vi "标定等待面板.vi"() -> ()   [LabVIEW 2013]
panel:
  in  "LVDT2ZADC":i64
  in  "LVDT2FADC":i64
  in  "LVDT1FADC":i64
  in  "LVDT1ZADC":i64
  in  "stop":bool
  # "标定中......"
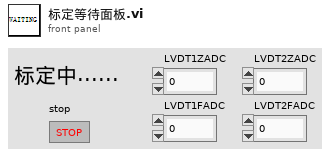
[diagram p1: front panel]
types:
  T1 = enum32{"DEH零度标定", "DEH满度标定", "阀门满度标定", "阀门零度标定", "最大正输出标定", "最大负输出标定", "零输出输出标定", "表头20mA标定", "表头4mA标定", "稳态偏差校准", "阀门位置自动标定", "转速4mA标定", "转速20mA标定"}
  T2 = cluster{"联机状态":bool, "外置清零信号":bool, "卡件工作模式":enum16{"无输出", "正常工作", "阀门常开", "阀门常闭"}, "卡件序列号":string, "卡件物理地址":string, "伺服阀输出电流CH1":dbl, "输出通道状态CH1":bool, "伺服阀输出电流CH2":dbl, "输出通道状态CH2":bool, "伺服输出使能CH1 ":bool, "伺服输出使能CH2":bool, "LVDT1类型":enum16{"未接入", "直流", "交流"}, "LVDT1直流回路":bool, "LVDT1次级线圈 2":bool, "LVDT1次级线圈 1":bool, "LVDT1初级线圈":bool, "LVDT2类型":enum16{"未接入", "直流", "交流"}, "LVDT2直流回路":bool, "LVDT2次级线圈 2":bool, "LVDT2次级线圈 1":bool, "LVDT2初级线圈":bool, "DEH回路状态":bool, "DEH类型":enum16{"内置", "外接"}, "转速反馈使能":bool, "LVDT1信号采样百分比":dbl, "LVDT2信号采样百分比":dbl, "DEH指令值":u8, "转速差反馈量":dbl, "回路1转速":dbl, "回路2转速":dbl, "回路3转速":dbl, "中选转速":dbl, "LVDT1 ADC":i16, "LVDT2 ADC":i16, "DEH ADC":i16, "LVDT1ZADC":i16, "LVDT2ZADC":i16, "LVDT1FADC":i16, "LVDT2FADC":i16, "DehZeroCali":bool, "DehFullCali":bool, "LVDT1ZeroCali":bool, "LVDT1FullCali":bool, "LVDT2ZeroCali":bool, "LVDT2FullCali":bool, "转速零度标定":i16, "转速满度标定":i16, "转速指令采样值":i16, "标准转速":dbl}
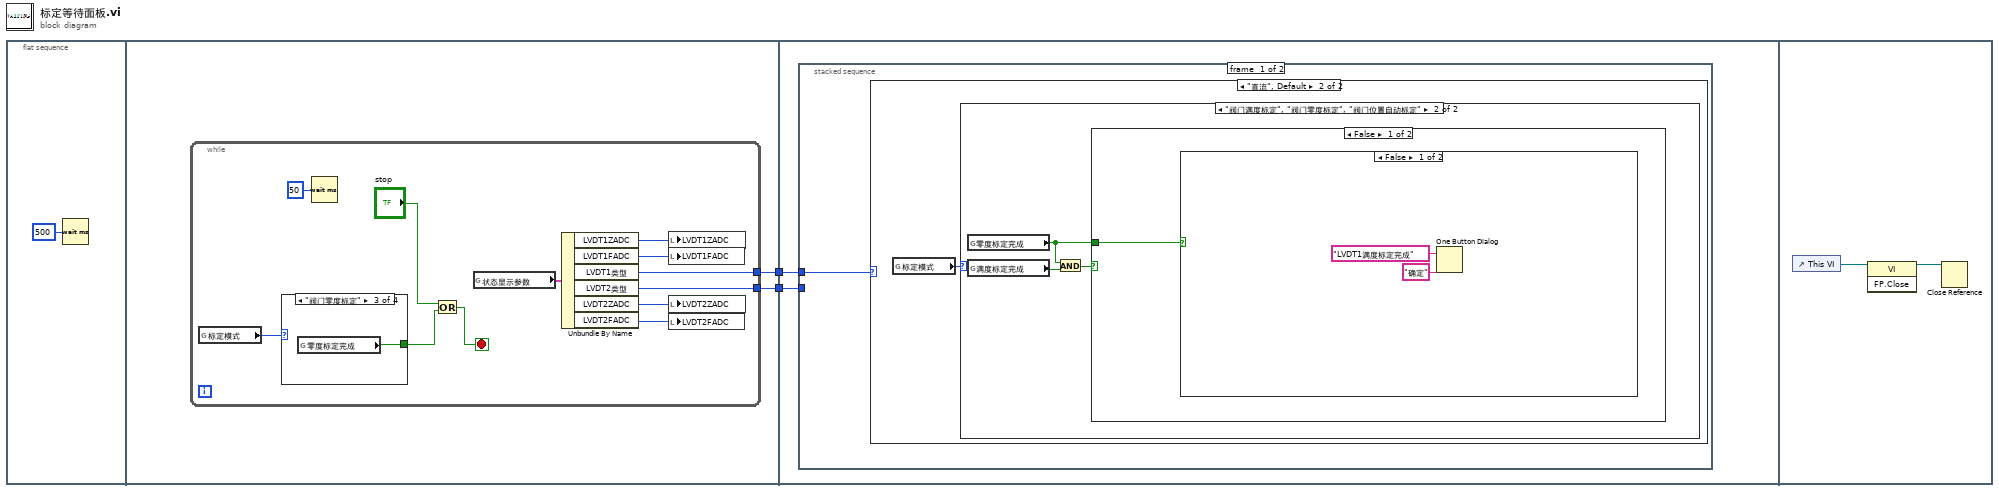
[diagram p0: block diagram]
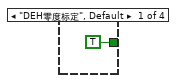
[diagram p2: hidden frame]
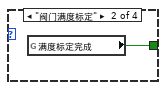
[diagram p3: hidden frame]
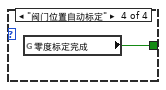
[diagram p4: hidden frame]
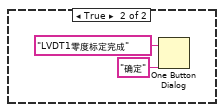
[diagram p7: hidden frame]
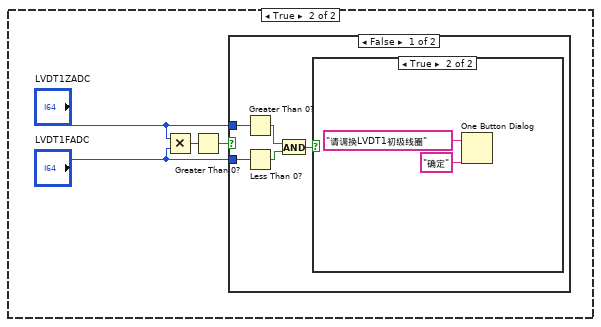
[diagram p8: hidden frame]
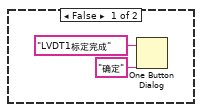
[diagram p9: hidden frame]
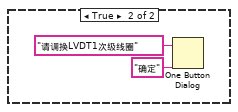
[diagram p10: hidden frame]
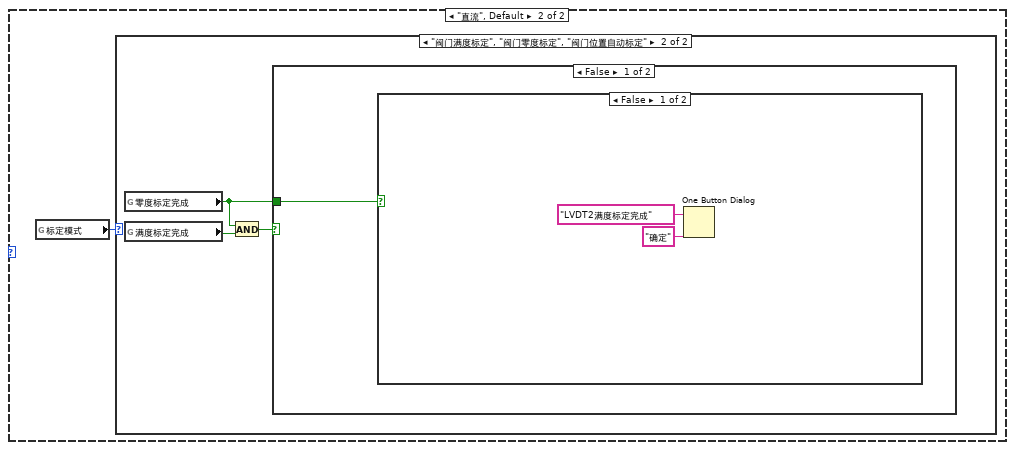
[diagram p12: hidden frame]
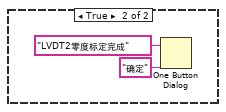
[diagram p14: hidden frame]
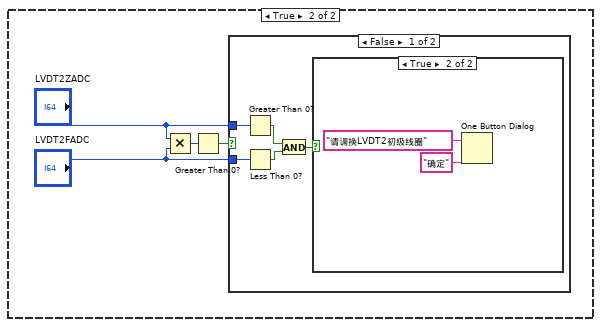
[diagram p15: hidden frame]
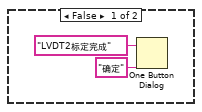
[diagram p16: hidden frame]
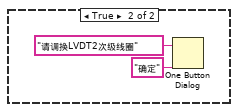
[diagram p17: hidden frame]
diagram:
  n1 = flat-sequence {
    tunnel: [w5] -> w2
    tunnel: [w4] -> w1
    tunnel: w2 -> [w23]
    tunnel: w1 -> [w22]
    frame #0 {
      n2 = Wait (ms)(milliseconds to wait=u32 500) -> ()  [unwired: 1 out]
    }
    frame #1 {
      n3 = while {
        tunnel: [w9] -> w5
        tunnel: [w8] -> w4
        stop <- w15 stop-if-true
        n4 = global read "标定模式.vi" "标定模式"() -> (w13:T1)
        n5 = case shown="\"阀门零度标定\"" w13 {
          tunnel: [TRUE ("标定完成") w19 w20 w21] -> w16
          frame "DEH零度标定", Default {
          }
          frame "阀门满度标定" {
            n6 = global read "满度标定完成.vi" "满度标定完成"() -> (w19:bool)
          }
          frame "阀门零度标定" {
            n7 = global read "零度标定完成.vi" "零度标定完成"() -> (w20:bool)
          }
          frame "阀门位置自动标定" {
            n8 = global read "零度标定完成.vi" "零度标定完成"() -> (w21:bool)
          }
        }
        n9 = Wait (ms)(milliseconds to wait=u32 50) -> ()  [unwired: 1 out]
        n10 = Or(x="stop", y=w16) -> (x .or. y?=w15:bool)
        n11 = global read "状态显示参数.vi" "状态显示参数"() -> (w12:T2)
        n12 = Unbundle By Name(w12) -> ("LVDT1ZADC"=w11:i16, "LVDT1FADC"=w10:i16, "LVDT1类型"=w9:enum16{"未接入", "直流", "交流"}, "LVDT2类型"=w8:enum16{"未接入", "直流", "交流"}, "LVDT2ZADC"=w7:i16, "LVDT2FADC"=w6:i16)
        n13 = local write "LVDT1ZADC"(w11) -> ()
        n14 = local write "LVDT1FADC"(w10) -> ()
        n15 = local write "LVDT2ZADC"(w7) -> ()
        n16 = local write "LVDT2FADC"(w6) -> ()
      }
    }
    frame #2 {
      n17 = stacked-sequence {
        tunnel: w23 -> [w24 _]
        tunnel: w22 -> [_ w49]
        frame #0 {
          n18 = case shown="\"直流\", Default" w24 {
            frame "未接入" {
            }
            frame "直流", Default {
              n19 = global read "标定模式.vi" "标定模式"() -> (w25:T1)
              n20 = case shown="\"阀门满度标定\", \"阀门零度标定\", \"阀门位置自动标定\"" w25 {
                frame "DEH零度标定", Default {
                }
                frame "阀门满度标定", "阀门零度标定", "阀门位置自动标定" {
                  n21 = global read "零度标定完成.vi" "零度标定完成"() -> (w26:bool)
                  n22 = global read "满度标定完成.vi" "满度标定完成"() -> (w28:bool)
                  n23 = And(x=w26, y=w28) -> (x .and. y?=w27:bool)
                  n24 = case shown="False" w27 {
                    tunnel: w26 -> [w29 _]
                    frame False {
                      n25 = case shown="False" w29 {
                        frame False {
                          n26 = One Button Dialog(message="LVDT1满度标定完成", button name ("OK")="确定") -> ()  [unwired: 1 out]
                        }
                        frame True {
                          n27 = One Button Dialog(message="LVDT1零度标定完成", button name ("OK")="确定") -> ()  [unwired: 1 out]
                        }
                      }
                    }
                    frame True {
                      n28 = Multiply(x="LVDT1ZADC", y="LVDT1FADC") -> (x*y=w37:i64)
                      n29 = Greater Than 0?(x=w37) -> (x > 0?=w36:bool)
                      n30 = case shown="False" w36 {
                        tunnel: "LVDT1FADC" -> [w39 _]
                        tunnel: "LVDT1ZADC" -> [w38 _]
                        frame False {
                          n31 = Greater Than 0?(x=w38) -> (x > 0?=w41:bool)
                          n32 = Less Than 0?(x=w39) -> (x < 0?=w40:bool)
                          n33 = And(x=w41, y=w40) -> (x .and. y?=w42:bool)
                          n34 = case shown="True" w42 {
                            frame False {
                              n35 = One Button Dialog(message="LVDT1标定完成", button name ("OK")="确定") -> ()  [unwired: 1 out]
                            }
                            frame True {
                              n36 = One Button Dialog(message="请调换LVDT1初级线圈", button name ("OK")="确定") -> ()  [unwired: 1 out]
                            }
                          }
                        }
                        frame True {
                          n37 = One Button Dialog(message="请调换LVDT1次级线圈", button name ("OK")="确定") -> ()  [unwired: 1 out]
                        }
                      }
                    }
                  }
                }
              }
            }
          }
        }
        frame #1 {
          n38 = case shown="\"未接入\"" w49 {
            frame "未接入" {
            }
            frame "直流", Default {
              n39 = global read "标定模式.vi" "标定模式"() -> (w50:T1)
              n40 = case shown="\"阀门满度标定\", \"阀门零度标定\", \"阀门位置自动标定\"" w50 {
                frame "DEH零度标定", Default {
                }
                frame "阀门满度标定", "阀门零度标定", "阀门位置自动标定" {
                  n41 = global read "零度标定完成.vi" "零度标定完成"() -> (w51:bool)
                  n42 = global read "满度标定完成.vi" "满度标定完成"() -> (w53:bool)
                  n43 = And(x=w51, y=w53) -> (x .and. y?=w52:bool)
                  n44 = case shown="False" w52 {
                    tunnel: w51 -> [w54 _]
                    frame False {
                      n45 = case shown="False" w54 {
                        frame False {
                          n46 = One Button Dialog(message="LVDT2满度标定完成", button name ("OK")="确定") -> ()  [unwired: 1 out]
                        }
                        frame True {
                          n47 = One Button Dialog(message="LVDT2零度标定完成", button name ("OK")="确定") -> ()  [unwired: 1 out]
                        }
                      }
                    }
                    frame True {
                      n48 = Multiply(x="LVDT2ZADC", y="LVDT2FADC") -> (x*y=w62:i64)
                      n49 = Greater Than 0?(x=w62) -> (x > 0?=w61:bool)
                      n50 = case shown="False" w61 {
                        tunnel: "LVDT2FADC" -> [w64 _]
                        tunnel: "LVDT2ZADC" -> [w63 _]
                        frame False {
                          n51 = Greater Than 0?(x=w63) -> (x > 0?=w66:bool)
                          n52 = Less Than 0?(x=w64) -> (x < 0?=w65:bool)
                          n53 = And(x=w66, y=w65) -> (x .and. y?=w67:bool)
                          n54 = case shown="True" w67 {
                            frame False {
                              n55 = One Button Dialog(message="LVDT2标定完成", button name ("OK")="确定") -> ()  [unwired: 1 out]
                            }
                            frame True {
                              n56 = One Button Dialog(message="请调换LVDT2初级线圈", button name ("OK")="确定") -> ()  [unwired: 1 out]
                            }
                          }
                        }
                        frame True {
                          n57 = One Button Dialog(message="请调换LVDT2次级线圈", button name ("OK")="确定") -> ()  [unwired: 1 out]
                        }
                      }
                    }
                  }
                }
              }
            }
          }
        }
      }
    }
    frame #3 {
      n58 = control-ref of="This VI"() -> (w75:refnum<vi>)
      n59 = invoke class="VI" method="FP.Close"(reference=w75) -> (reference out=w74:refnum<vi>)  [unwired: 2 in, 2 out]
      n60 = Close Reference(reference=w74) -> ()  [unwired: 1 in, 1 out]
    }
  }
